vi "observacao.vi"() -> ()   [LabVIEW 2012] (continued)
            # "MUDANÇA:\nBit EMBREAGEM trocado pelos bits RAPIDO e LIGEIRO para detectar a retirada do objeto da posição centrada."
            # "MUDANÇA FUTURA:\nTrocar globais de calagem por valores \"latch\" dessas globais. Finalidade: manter display de coordenadas consistentes mesmo quando o usuário zerar as calagens, especialmente a local, para o próximo apontamento."
            # "ATUALIZA INDICADORES DO PAINEL"
            n267 = local read "ChkCalGlobal"() -> (w274:bool)
            n268 = global read "Global_Telescopio.vi" "PosDEC"() -> (w277:dbl)
            n269 = global read "Global_Telescopio.vi" "Sideral Time"() -> (w279:dbl)
            n270 = global read "Global_Telescopio.vi" "ObjCentrado"() -> (w250:bool)
            "ObjCentrado" <- w250
            n271 = global read "Global_Telescopio.vi" "PosAH"() -> (w278:dbl)
            n272 = call "Calcula epoch.vi"() -> ("epoch"=→"Epoch":dbl)  [unwired: 2 in]
            n273 = call "Bit Status AH.vi"("NomeStatus"=w263) -> ("StatBit"=w261:bool)
            n274 = call "Bit Status AH.vi"("NomeStatus"=w258) -> ("StatBit"=w257:bool)
            n275 = call "Bit Status DEC.vi"("NomeStatus"=w262) -> ("StatBit"=w255:bool)
            n276 = call "Bit Status DEC.vi"("NomeStatus"=w259) -> ("StatBit"=w256:bool)
            n277 = Compound Arithmetic op=OR(w261, w257, w255, w256) -> (w260:bool)
            n278 = case shown="True" w260 {
              frame False {
              }
              frame True {
                n279 = global write "Global_Telescopio.vi" "ObjCentrado"(FALSE) -> ()
              }
            }
            n280 = Tick Count (ms)() -> (millisecond timer value=w246:u32)
            n281 = local read "LedPointing"() -> (w245:bool)
            n282 = case shown="True" w250 {
              tunnel: [w356 w373] -> w271
              tunnel: [w355 w372] -> w267
              tunnel: [w358 w376] -> w251
              tunnel: [w357 w374] -> w264
              tunnel: w279 -> [w356 w373]
              tunnel: w278 -> [w361 _]
              tunnel: w277 -> [w360 _]
              tunnel: w274 -> [w359 _]
              tunnel: [w354 w370] -> _
              tunnel: w246 -> [w354 w370]
              frame False {
                n283 = case shown="False" w359 {
                  tunnel: w360 -> [w363 w369]
                  tunnel: [w363 w368] -> w358
                  tunnel: w361 -> [w362 w367]
                  tunnel: [w362 w364] -> w357
                  frame False {
                  }
                  frame True {
                    n284 = global read "Global_Telescopio.vi" "Calagem AH"() -> (w365:dbl)
                    n285 = global read "Global_Telescopio.vi" "Calagem DEC"() -> (w366:dbl)
                    n286 = Subtract(x=w367, y=w365) -> (x-y=w364:dbl)
                    n287 = Subtract(x=w369, y=w366) -> (x-y=w368:dbl)
                  }
                }
                n288 = Subtract(x=w356, y=w357) -> (x-y=w355:dbl)
              }
              frame True {
                # "PROCESSO PRECESSÃO"
                n289 = local read "Temp amb"() -> (w379:string)
                n290 = local read "hum local"() -> (w377:string)
                n291 = local read "MeanDEC"() -> (w380:string)
                n292 = local read "pressão atm"() -> (w378:string)
                n293 = local read "PM_RA"() -> (w375:string)
                n294 = local read "MeanRA"() -> (w381:string)
                n295 = local read "PM_DEC"() -> (w371:string)
                n296 = call "PrecessFortran.vi"("Asc reta"=w381, "Var RA"=w375, "Declinação"=w380, "Temperatura (Kelvin)"=w379, "Pressao atmosferica (mB)"=w378, "Humidade relativa (0 a 1)"=w377, "Var DEC"=w371) -> ("Observed RA (radians)"=w372:dbl, "Observed Dec (radians)"=w376:dbl)  [unwired: 2 in, 5 out]
                n297 = Subtract(x=w373, y=w372) -> (x-y=w374:dbl)
              }
            }
            "AtualDEC" <- w251
            n298 = case shown="True" w250 {
              tunnel: w251 -> [_ w310]
              tunnel: [w307 w309] -> w276
              tunnel: [w307 w308] -> w275
              frame False {
                w307 = 0.0
              }
              frame True {
                n299 = stacked-sequence {
                  seq-local: [w311 _ _] -> [_ _ w349]
                  tunnel: w310 -> [_ w318 _]
                  tunnel: [_ w317 _] -> w309
                  tunnel: [_ w316 _] -> w308
                  frame #0 {
                    n300 = Tick Count (ms)() -> (millisecond timer value=w311:u32)
                  }
                  frame #1 {
                    w319 = u16 3 items=["Alarme", "Atencao", "Erro", "Ocupado", "Protecao", "Embreagem", "Tracking", "Var. Track", "Rápido", "Ligeiro", "Médio", "Lento", "Em movimento", ""] ("NomeStatus")
                    w320 = u16 3 items=["Alarme", "Atencao", "Erro", "Ocupado", "Protecao", "Embreagem", "Tracking", "Var. Track", "Rápido", "Ligeiro", "Médio", "Lento", "Em movimento", ""] ("NomeStatus")
                    # "PROCESSO LEITURA POS_MOTOR"
                    n301 = local read "MOV_IDX_AH"() -> (w314:bool)
                    n302 = local read "MOV_IDX_DEC"() -> (w312:bool)
                    n303 = call "Bit Status AH.vi"("NomeStatus"=w320) -> ("StatBit"=w315:bool)
                    n304 = call "Bit Status DEC.vi"("NomeStatus"=w319) -> ("StatBit"=w313:bool)
                    n305 = case shown="False" w315 {
                      tunnel: w318 -> [w334 _]
                      tunnel: [w333 w348] -> w317
                      tunnel: w314 -> [w332 _]
                      frame False {
                        n306 = case shown="False" w332 {
                          tunnel: w334 -> [w342 _]
                          tunnel: [w338 w347] -> w333
                          frame False {
                            w345 = u16 1 items=["ZERO", "AH", "DEC", "TUBO", "CUP"] ("Controlador")
                            # "RA"
                            # "AH"
                            n307 = call "Get Posic Motor Indexer.vi"("Controlador"=w345) -> ("PosMotor"=w336:dbl)
                            n308 = global read "Global_Telescopio.vi" "AcumPrecRA"() -> (w339:dbl)
                            n309 = Negate(x=w336) -> (-x=w337:dbl)
                            n310 = Subtract(x=w337, y=w339) -> (x-y=w346:dbl)
                            n311 = global read "Global_Telescopio.vi" "AcumAG RA"() -> (w340:dbl)
                            n312 = Cosine(x=w342) -> (cos(x)=w341:dbl)
                            n313 = Absolute Value(x=w341) -> (abs(x)=w335:dbl)
                            n314 = Subtract(x=w346, y=w340) -> (x-y=w344:dbl)
                            n315 = Multiply(x=w335, y=w344) -> (x*y=w343:dbl)
                            n316 = call "Rad to Arcsec.vi"("Radiano"=w343) -> ("Arcsec"=w338:dbl)
                          }
                          frame True {
                            n317 = local read "Offset RA"() -> (w347:dbl)
                          }
                        }
                      }
                      frame True {
                        n318 = local read "Offset RA"() -> (w348:dbl)
                      }
                    }
                    n319 = case shown="False" w313 {
                      tunnel: [w322 w331] -> w316
                      tunnel: w312 -> [w321 _]
                      frame False {
                        n320 = case shown="False" w321 {
                          tunnel: [w323 w330] -> w322
                          frame False {
                            w326 = u16 2 items=["ZERO", "AH", "DEC", "TUBO", "CUP"] ("Controlador")
                            n321 = call "Get Posic Motor Indexer.vi"("Controlador"=w326) -> ("PosMotor"=w328:dbl)
                            n322 = global read "Global_Telescopio.vi" "AcumPrecDEC"() -> (w324:dbl)
                            n323 = Subtract(x=w328, y=w324) -> (x-y=w329:dbl)
                            n324 = global read "Global_Telescopio.vi" "AcumAG DEC"() -> (w325:dbl)
                            n325 = Subtract(x=w329, y=w325) -> (x-y=w327:dbl)
                            n326 = call "Rad to Arcsec.vi"("Radiano"=w327) -> ("Arcsec"=w323:dbl)
                          }
                          frame True {
                            n327 = local read "Offset DEC"() -> (w330:dbl)
                          }
                        }
                      }
                      frame True {
                        n328 = local read "Offset DEC"() -> (w331:dbl)
                      }
                    }
                  }
                  frame #2 {
                    n329 = flat-sequence {
                      tunnel: w349 -> [w350]
                      frame #0 {
                        n330 = Tick Count (ms)() -> (millisecond timer value=w351:u32)
                        n331 = Subtract(x=w351, y=w351) -> (x-y=→"dtAUX2":u32)
                        n332 = Subtract(x=w351, y=w350) -> (x-y=→"dtAUX3":u32)
                      }
                    }
                  }
                }
              }
            }
            "Offset RA" <- w276
            "Offset DEC" <- w275
            n333 = case shown="False" w245 {
              frame False {
                w285 = 0
                n334 = property on="BtPointPrecess" class="Bool"("DisabledEnum"=w285) -> ()  [unwired: 2 in, 2 out]
                n335 = property on="BtPointObjClear" class="Bool"("DisabledEnum"=w285) -> ()  [unwired: 2 in, 2 out]
              }
              frame True {
                w286 = 2
                n336 = property on="BtPointPrecess" class="Bool"("DisabledEnum"=w286) -> ()  [unwired: 2 in, 2 out]
                n337 = property on="BtPointObjClear" class="Bool"("DisabledEnum"=w286) -> ()  [unwired: 2 in, 2 out]
              }
            }
            n338 = call "Normliza_AH.vi"("PosAH"=w264) -> ("Numeric"=w249:dbl)
            n339 = Add(x=w269, y=w267) -> (x+y=w268:dbl)
            n340 = Add(x=w269, y=w271) -> (x+y=w272:dbl)
            n341 = Less Than 0?(x=w271) -> (x < 0?=w273:bool)
            n342 = Less Than 0?(x=w267) -> (x < 0?=w270:bool)
            n343 = Select(t=w272, s=w273, f=w271) -> (s? t:f=w252:dbl)
            n344 = Select(t=w268, s=w270, f=w267) -> (s? t:f=w253:dbl)
            n345 = case shown="True" w250 {
              tunnel: ["" w294] -> w254
              tunnel: w253 -> [_ w291]
              tunnel: w252 -> [_ w292]
              tunnel: w251 -> [_ w293]
              frame False {
              }
              frame True {
                n346 = disable-structure shown="Disabled" {
                  disable-tunnel: w293 -> [w305 _]
                  disable-tunnel: w292 -> [w304 _]
                  disable-tunnel: w291 -> [w303 _]
                  disable-tunnel: [w302 _] -> _
                  frame Disabled {
                    n347 = call "Hora_Limite.vi"("Asc Reta RA rad"=w303, "Sideral Time rad"=w304, "Declinação rad"=w305) -> ("TO Tempo de Observação Horas"=w302:dbl)  [unwired: 2 in]
                  }
                  frame Enabled {
                  }
                }
                n348 = call "Novo_tempo_obs.vi"() -> ("TO rad"=w289:dbl)  [unwired: 10 in, 1 out]
                n349 = Greater Than 0?(x=w289) -> (x > 0?=w288:bool)
                n350 = case shown="True" w288 {
                  tunnel: [w296 w299] -> w290
                  tunnel: w289 -> [w296 w298]
                  frame False {
                  }
                  frame True {
                    n351 = Random Number (0-1)() -> (number: 0 to 1=w300:dbl)
                    n352 = Multiply(x=w300, y=7.27e-05) -> (x*y=w297:dbl)
                    n353 = Add(x=w298, y=w297) -> (x+y=w299:dbl)
                  }
                }
                n354 = call "rad_hms.vi"("TRUE=HORA\nFALSE=GRAU"=TRUE ("TRUE=HORA\nFALSE=GRAU"), "Radiano"=w290) -> ("Hora/Graus Texto Decimal"=w294:string)  [unwired: 3 in]
              }
            }
            "Time to Limit" <- w254
            n355 = call "rad_hms.vi"("TRUE=HORA\nFALSE=GRAU"=TRUE ("TRUE=HORA\nFALSE=GRAU"), "Radiano"=w252) -> ("Hora/Graus Texto Decimal"=w266:string)  [unwired: 3 in]
            "Sideral time" <- w266
            n356 = call "rad_hms.vi"("TRUE=HORA\nFALSE=GRAU"=TRUE, "Radiano"=w253) -> ("Hora/Graus Texto Decimal"=w265:string)  [unwired: 3 in]
            "Right Ascention" <- w265
            n357 = call "rad_hms.vi"("TRUE=HORA\nFALSE=GRAU"=TRUE, "Radiano"=w249) -> ("Hora/Graus Texto Decimal"=w248:string)  [unwired: 3 in]
            "Hour Angle" <- w248
            "Hour Angle 2" <- w248
            n358 = call "rad_hms.vi"("TRUE=HORA\nFALSE=GRAU"=FALSE, "Radiano"=w251) -> ("Hora/Graus Texto Decimal"=w247:string)  [unwired: 3 in]
            "Declination" <- w247
            "DEC" <- w247
            n359 = global write "Global_Telescopio.vi" "Right Ascention"(w265) -> ()
            n360 = global write "Global_Telescopio.vi" "Hour Angle"(w248) -> ()
            n361 = global write "Global_Telescopio.vi" "Sideral time"(w266) -> ()
            n362 = global write "Global_Telescopio.vi" "Declination"(w247) -> ()
            n363 = global write "Global_Telescopio.vi" "AH_now"(w249) -> ()
            n364 = global write "Global_Telescopio.vi" "delta_now"(w251) -> ()
          }
          frame #2 {
            w406 = -0.39330025  # LatOPD rad
            # "ALTERAÇÃO FEITA EM 12/12/2012\nFEITA PARA RESOLVER EXCESSÍVOS\nMOVIMENTOS DO ACOMP.SID. DA\nCÚPULA (DANIEL). A condição de statCUP=0 foi inserida em 08/5/2013-> Só corrige a cúpula se esta estiver parada!"
            # "Horas"
            # "MUDANÇA FUTURA:\nPassar LatOPD para Global"
            # "az"
            # "z"
            # "Cálculo do Azimute da Cúpula e Hab Acompanham. Cúpula"
            # "Lógica de Segurança"
            # "ANGULO ZENITAL"
            n365 = global read "Global_Telescopio.vi" "OffsetCupula"() -> (w415:dbl)
            n366 = global read "Global_Telescopio.vi" "AH_now"() -> (w397:dbl)
            n367 = global read "Global_Telescopio.vi" "delta_now"() -> (w405:dbl)
            n368 = global read "Global_Telescopio.vi" "ErroMaxCup"() -> (w384:i16)
            n369 = global read "Global_Telescopio.vi" "Limite EAST"() -> (w398:dbl)
            n370 = global read "Global_Telescopio.vi" "Limite WEST"() -> (w399:dbl)
            n371 = global read "Global_Telescopio.vi" "PosCUP"() -> (w385:i16)
            "PosCUP" <- w385
            n372 = local read "Tick Cupula"() -> (w389:u32)
            n373 = call "Calculo_do_Azimute_da_Cupula_2.vi"("AH"=w397, "DEC"=w405, "OffsetTCSPD"=w415) -> ("PosCup"=w382:u16)  [unwired: 3 in, 1 out]
            "Azimute cup" <- w382
            n374 = Tick Count (ms)() -> (millisecond timer value=w390:u32)
            n375 = Multiply(x=w397, y=3.8197) -> (x*y=w400:dbl)
            n376 = call "Altura_e_Azimute.vi"("LAT rad"=w406, "DEC rad"=w405, "AH rad"=w397) -> ("AZIMUTE graus"=w403:dbl, "ANG. ZENITAL graus"=w404:dbl, "AZIMUTE rad"=w407:dbl, "ANG. ZENITAL rad"=w408:dbl)  [unwired: 2 out]
            "Azimuth" <- w403
            "Zenital angle" <- w404
            n377 = Greater Or Equal?(x=w390, y=w389) -> (x >= y?=w388:bool)
            n378 = Greater?(x=w400, y=w398) -> (0:w396:bool)
            n379 = Less?(x=w400, y=w399) -> (x < y?=w395:bool)
            n380 = call "Verifica_Correcao_CUP.vi"("Erro max"=w384, "Pos Atual"=w385, "Azimute"=w382) -> ("Corrigir?"=w383:bool)  [unwired: 2 in]
            n381 = Not And(1:w395, 2:w396) -> (0:w392:bool)
            n382 = local read "statCUP"() -> (w387:i32)
            n383 = call "Calcula_Proteção.vi"("Zenital angle rad"=w408, "Azimute rad"=w407) -> ("Z_SEGURANÇA_GRAUS"=w417:dbl, "Prot Segur"=w419:bool, "Z_LIBERA_GRAUS"=w416:dbl, "Z_MAX_GRAUS"=w418:dbl, "Prot Zmax"=w393:bool)
            n384 = Equal To 0?(x=w387) -> (x = 0?=w386:bool)
            n385 = global write "Global_Telescopio.vi" "Z_SEGURANÇA_GRAUS"(w417) -> ()
            n386 = global write "Global_Telescopio.vi" "Zenital angle GRAUS"(w404) -> ()
            n387 = global write "Global_Telescopio.vi" "Azimute GRAUS"(w403) -> ()
            n388 = global write "Global_Telescopio.vi" "Z_MAX_GRAUS"(w418) -> ()
            n389 = global write "Global_Telescopio.vi" "Z_LIBERA_GRAUS"(w416) -> ()
            n390 = Compound Arithmetic op=AND(w383, "DOME", w388, w386) -> (w414:bool)
            n391 = case shown="True" w414 {
              tunnel: w382 -> [_ w428]
              tunnel: FALSE -> [_ w426]
              frame False {
              }
              frame True {
                # "TEMPO CÚPULA"
                # "2m Tempo para novo movimento"
                n392 = local write "Dome on Target"(w426) -> ()
                n393 = Tick Count (ms)() -> (millisecond timer value=w425:u32)
                n394 = To Word Integer(number=w428) -> (16bit integer=w422:i16)
                n395 = local write "statCUP"(1 ("statCUP")) -> ()
                n396 = Add(x=w425, y=u32 120000) -> (x+y=→"Tick Cupula":u32)
                n397 = global write "Global_Telescopio.vi" "TargetCUP"(w422) -> ()
              }
            }
            n398 = Or(x=w392, y=w393) -> (x .or. y?=w394:bool)
            n399 = global read "Global_Telescopio.vi" "LIMITE"() -> (w413:bool)
            n400 = Or(x=w413, y=w394) -> (x .or. y?=w412:bool)
            "Proteção" <- w412
            n401 = call "Borda_Subida_Segurança.vi"("Entrada"=w419) -> ("Boolean"=w420:bool)
            n402 = call "Borda_Subida_Z_max.vi"("Entrada"=w412) -> ("Boolean"=w421:bool)
            n403 = Select(t=u8 2 ("Disabled"), s=w412, f=u8 0 ("Disabled")) -> (s? t:f=w409:u8)
            n404 = property on="MOUNT" class="Bool (strict)"("Disabled"=w409) -> ()  [unwired: 2 in, 2 out]
            n405 = case shown="True" w420 {
              frame False {
              }
              frame True {
                w431 = u16 2 items=["ZERO", "AH", "DEC", "TUBO", "CUP"] ("Controlador")
                w430 = "FREAR" ("Comando")
                w432 = u16 1 items=["ZERO", "AH", "DEC", "TUBO", "CUP"] ("Controlador")
                w429 = "EIXO" ("Dispositivo")
                n406 = call "Monta Comando.vi"("Comando"=w430, "Dispositivo"=w429, "Controlador"=w432) -> ()  [unwired: 4 in, 3 out]
                n407 = call "Monta Comando.vi"("Comando"=w430, "Dispositivo"=w429, "Controlador"=w431) -> ()  [unwired: 4 in, 3 out]
              }
            }
            n408 = case shown="True" w421 {
              frame False {
              }
              frame True {
                w435 = FALSE
                w433 = "Telescópio parado por inclinação excessiva!" ("SYSTEM MESSAGES")
                n409 = local write "LED MOUNT"(w435) -> ()
                n410 = local write "MOUNT"(w435) -> ()
                n411 = global write "Global_Telescopio.vi" "ObjCentrado"(FALSE) -> ()
                n412 = global write "Global_Telescopio.vi" "STOP ALL"(TRUE ("STOP ALL")) -> ()
                n413 = call "Monta_Mensagem.vi"("Mensagem"=w433) -> ()  [unwired: 2 in]
                n414 = call "Salva_systems_messages.vi"("Mensagem"=w433) -> ()  [unwired: 5 in]
              }
            }
            "Led Chave Dome" <- "DOME"
          }
          frame #3 {
            w442 = u32 500 ("millisecond multiple")
            w456 = u16 3 items=["Alarme", "Atencao", "Erro", "Ocupado", "TBD", "LCB", "Trapeira", "Paravento", "DomoRap", "DomoCW", "DomoCCW", "TBD", "Em movimento", "TBD"] ("NomeStatus")
            w470 = u16 3 items=["Alarme", "Atencao", "Erro", "Ocupado", "Protecao", "Embreagem", "Tracking", "Var. Track", "Rápido", "Ligeiro", "Médio", "Lento", "Em movimento", ""] ("NomeStatus")
            w471 = u16 3 items=["Alarme", "Atencao", "Erro", "Ocupado", "Protecao", "Embreagem", "Tracking", "Var. Track", "Rápido", "Ligeiro", "Médio", "Lento", "Em movimento", ""] ("NomeStatus")
            # "04-07-2022\nValor de Erro PROTEC\nalterado de 5 para 10"
            # "MUDANÇA: \nIncluído CASE"
            # "Esse metrônomo determina\no ciclo de 0,5 segundo dos\ncálculos rápidos e totais!"
            # "PROCESSO APONTAMENTO"
            # "MÁQUINA DE ESTADO DO APONTAMENTO"
            # "Seta nome para GO/STOP"
            n415 = global read "Global_Telescopio.vi" "LimiarRapMed"() -> (w472:dbl)
            n416 = global write "Global_Telescopio.vi" "Estado DEC"("statDEC") -> ()
            n417 = global read "Global_Telescopio.vi" "Sideral Time"() -> (w450:dbl)
            n418 = global read "Global_Telescopio.vi" "PosAH"() -> (w475:dbl)
            n419 = global read "Global_Telescopio.vi" "ErroMaxEixo"() -> (w459:dbl)
            n420 = global read "Global_Telescopio.vi" "PosDEC"() -> (w473:dbl)
            n421 = global read "Global_Telescopio.vi" "TargetRA"() -> (w476:dbl)
            n422 = global read "Global_Telescopio.vi" "TargetDEC"() -> (w474:dbl)
            n423 = call "Bit Status DEC.vi"("NomeStatus"=w470) -> ("StatBit"=w458:bool)
            n424 = call "Bit Status AH.vi"("NomeStatus"=w471) -> ("StatBit"=w457:bool)
            n425 = case shown="4" "statDEC" {
              selector: "statDEC" -> [w605 _ _ _ _ _ _ _ _]
              tunnel: [w605 w612 w642 w664 w691 w715 0 ("t") w732 w737] -> w451
              tunnel: w474 -> [_ w611 _ w658 _ _ _ _ _]
              tunnel: w473 -> [_ w607 _ w661 _ _ _ _ _]
              tunnel: w459 -> [_ _ _ w662 _ _ _ _ _]
              tunnel: w472 -> [_ w613 _ _ _ _ _ _ _]
              tunnel: w458 -> [_ w610 _ w657 _ _ _ _ _]
              frame 0, Default {
                w603 = 0 ("CR DEC")
                # "Sem apontamento"
                n426 = call "TickTimeout.vi"() -> ("msTick"=→"TimeoutDEC":u32)  [unwired: 2 in, 2 out]
                n427 = local write "CR DEC"(w603) -> ()
                n428 = local write "C. DEC"(w603) -> ()
              }
              frame 1 {
                # "Envia\nComando"
                n429 = Subtract(x=w611, y=w607) -> (x-y=w609:dbl)
                n430 = Absolute Value(x=w609) -> (abs(x)=w614:dbl)
                n431 = Less?(x=w614, y=w613) -> (x < y?=w608:bool)
                n432 = case shown="False" w608 {
                  tunnel: [w618 3] -> w612
                  tunnel: w611 -> [w617 _]
                  tunnel: w609 -> [w616 _]
                  tunnel: w610 -> [w615 _]
                  frame False {
                    # "destino"
                    # "Fora do"
                    n433 = case shown="False" w615 {
                      tunnel: [w622 w630] -> w618
                      tunnel: w617 -> [w625 _]
                      tunnel: w616 -> [_ _]
                      frame False {
                        w629 = u16 2 items=["ZERO", "AH", "DEC", "TUBO", "CUP"] ("Controlador")
                        # "limpa flag"
                        # "CLP Pronto"
                        n434 = local write "Flag ativo DEC"(FALSE ("Flag ativo DEC")) -> ()
                        n435 = call "rad_hms.vi"("TRUE=HORA\nFALSE=GRAU"=FALSE, "Radiano"=w625) -> ("Hora/Graus Texto Decimal"=w626:string)  [unwired: 3 in]
                        n436 = call "Monta Comando.vi"("Set Point"=w626, "Comando"="MOVER_RAP", "Dispositivo"="EIXO" ("Comando"), "Controlador"=w629) -> ("Erro Comunicação"=w620:bool)  [unwired: 3 in, 2 out]
                        n437 = Select(t=6, s=w620, f=20) -> (s? t:f=w622:i32)
                      }
                      frame True {
                        # "CLP Ocupado"
                        n438 = local read "TimeoutDEC"() -> (w632:u32)
                        n439 = call "TickTimeout.vi"("msInicial"=w632, "msTimeout"=u32 4000) -> ("Timeout"=w631:bool)  [unwired: 2 out]
                        n440 = case shown="False" w631 {
                          tunnel: [1 5] -> w630
                          frame False {
                          }
                          frame True {
                            # "Tratar\nTimeout"
                          }
                        }
                      }
                    }
                  }
                  frame True {
                    # "Dist. pequena p/ mov. rápido"
                    # "Ligar mov. lento"
                    n441 = call "TickTimeout.vi"() -> ("msTick"=w636:u32)  [unwired: 2 in, 2 out]
                    n442 = local write "TimeoutDEC"(w636) -> ()
                  }
                }
                n443 = local write "dec="(FALSE ("dec=")) -> ()
              }
              frame 2 {
                w643 = u16 12 items=["Alarme", "Atencao", "Erro", "Ocupado", "Protecao", "Embreagem", "Tracking", "Var. Track", "Rápido", "Ligeiro", "Médio", "Lento", "Em movimento", ""] ("NomeStatus")
                # "Aguarda fim mov. Rap."
                n444 = call "Bit Status DEC.vi"("NomeStatus"=w643) -> ("StatBit"=w644:bool)
                n445 = case shown="True" w644 {
                  tunnel: [1 w653] -> w641
                  frame False {
                    # "Motor parado.\nTestar se chegou\nao destino"
                    n446 = call "TickTimeout.vi"() -> ("msTick"=w649:u32)  [unwired: 2 in, 2 out]
                    n447 = local write "TimeoutDEC"(w649) -> ()
                  }
                  frame True {
                    # "Ainda movendo...\nAGUARDAR"
                    n448 = local read "Erro PROTEC"() -> (w655:i32)
                    n449 = call "PROTECAO_DEC.vi"() -> ("CONT DEC"=w656:i32)  [unwired: 11 in]
                    "C. DEC" <- w656
                    n450 = Greater Or Equal?(x=w656, y=w655) -> (x >= y?=w651:bool)
                    n451 = Select(t=6, s=w651, f=2) -> (s? t:f=w653:i32)
                  }
                }
                n452 = global read "Global_Telescopio.vi" "Habilita supervisao"() -> (w639:bool)
                n453 = case shown="True" w639 {
                  tunnel: [FALSE w648] -> w638
                  frame False {
                  }
                  frame True {
                    n454 = local read "Erro Lim"() -> (w646:i32)
                    n455 = Greater Or Equal?(x="CR DEC", y=w646) -> (x >= y?=w648:bool)
                  }
                }
                n456 = Select(t=6, s=w638, f=w641) -> (s? t:f=w642:i32)
              }
              frame 3 {
                # "Mov.Lento"
                n457 = Subtract(x=w658, y=w661) -> (x-y=w659:dbl)
                n458 = Absolute Value(x=w659) -> (abs(x)=w663:dbl)
                n459 = Less Or Equal?(x=w663, y=w662) -> (x <= y?=w660:bool)
                n460 = case shown="False" w660 {
                  selector: w660 -> [_ w687]
                  tunnel: [w666 0] -> w664
                  tunnel: w659 -> [w665 _]
                  tunnel: w658 -> [_ w686]
                  tunnel: w657 -> [w667 _]
                  frame False {
                    n461 = case shown="False" w667 {
                      tunnel: [w671 w680] -> w666
                      tunnel: w665 -> [w674 _]
                      frame False {
                        w679 = u16 2 items=["ZERO", "AH", "DEC", "TUBO", "CUP"] ("Controlador")
                        # "limpa flag"
                        # "Mov. lento"
                        n462 = call "TickTimeout.vi"() -> ("msTick"=w673:u32)  [unwired: 2 in, 2 out]
                        n463 = local write "TimeoutDEC"(w673) -> ()
                        n464 = call "rad_hms.vi"("TRUE=HORA\nFALSE=GRAU"=FALSE ("TRUE=HORA\nFALSE=GRAU"), "Radiano"=w674) -> ("Hora/Graus Texto Decimal"=w676:string)  [unwired: 3 in]
                        n465 = local write "Flag ativo DEC"(FALSE ("Flag ativo DEC")) -> ()
                        n466 = call "Monta Comando.vi"("Set Point"=w676, "Comando"="MOVER_REL", "Dispositivo"="EIXO" ("Comando"), "Controlador"=w679) -> ("Erro Comunicação"=w669:bool)  [unwired: 3 in, 2 out]
                        n467 = Select(t=6, s=w669, f=40) -> (s? t:f=w671:i32)
                      }
                      frame True {
                        # "CLP Ocupado"
                        n468 = local read "TimeoutDEC"() -> (w682:u32)
                        n469 = call "TickTimeout.vi"("msInicial"=w682, "msTimeout"=u32 2000) -> ("Timeout"=w681:bool)  [unwired: 2 out]
                        n470 = case shown="False" w681 {
                          tunnel: [3 5] -> w680
                          frame False {
                          }
                          frame True {
                          }
                        }
                      }
                    }
                  }
                  frame True {
                    # "DEC no destino"
                    n471 = local write "LatchDeslocDEC"(w686) -> ()
                    "DEC on Target" <- w687
                  }
                }
              }
              frame 4 {
                w694 = u16 12 items=["Alarme", "Atencao", "Erro", "Ocupado", "Protecao", "Embreagem", "Tracking", "Var. Track", "Rápido", "Ligeiro", "Médio", "Lento", "Em movimento", ""] ("NomeStatus")
                # "Aguarda fim mov. lento"
                n472 = call "Bit Status DEC.vi"("NomeStatus"=w694) -> ("StatBit"=w695:bool)
                n473 = case shown="True" w695 {
                  tunnel: [3 w705] -> w690
                  frame False {
                    # "Motor parado.\nTestar se chegou\nao destino"
                    n474 = call "TickTimeout.vi"() -> ("msTick"=w700:u32)  [unwired: 2 in, 2 out]
                    n475 = local write "TimeoutDEC"(w700) -> ()
                  }
                  frame True {
                    n476 = local read "Erro PROTEC"() -> (w707:i32)
                    n477 = call "PROTECAO_DEC.vi"() -> ("CONT DEC"=w702:i32)  [unwired: 11 in]
                    n478 = local write "C. DEC"(w702) -> ()
                    n479 = Greater Or Equal?(x=w702, y=w707) -> (x >= y?=w704:bool)
                    n480 = local read "TimeoutDEC"() -> (w709:u32)
                    n481 = call "TickTimeout.vi"("msInicial"=w709, "msTimeout"=u32 4000) -> ("Timeout"=w708:bool)  [unwired: 2 out]
                    n482 = case shown="False" w708 {
                      tunnel: [4 5] -> w703
                      frame False {
                      }
                      frame True {
                      }
                    }
                    n483 = Select(t=6, s=w704, f=w703) -> (s? t:f=w705:i32)
                  }
                }
                n484 = global read "Global_Telescopio.vi" "Habilita supervisao"() -> (w692:bool)
                n485 = case shown="True" w692 {
                  tunnel: [FALSE w699] -> w689
                  frame False {
                  }
                  frame True {
                    n486 = local read "CR DEC"() -> (w698:i32)
                    n487 = local read "Erro Lim"() -> (w697:i32)
                    n488 = Greater Or Equal?(x=w698, y=w697) -> (x >= y?=w699:bool)
                  }
                }
                n489 = Select(t=6, s=w689, f=w690) -> (s? t:f=w691:i32)
              }
              frame 5 {
                w720 = u16 2 items=["ZERO", "AH", "DEC", "TUBO", "CUP"] ("Controlador")
                # "Reiniciar apontamento"
                # "Trata Timeout"
                n490 = call "TickTimeout.vi"() -> ("msTick"=w717:u32)  [unwired: 2 in, 2 out]
                n491 = local write "TimeoutDEC"(w717) -> ()
                n492 = call "Monta Comando.vi"("Comando"="PARAR", "Dispositivo"="PROG" ("Comando"), "Controlador"=w720) -> ("Erro Comunicação"=w713:bool)  [unwired: 4 in, 2 out]
                n493 = Select(t=6, s=w713, f=1) -> (s? t:f=w715:i32)
              }
              frame 6 {
                # "PARADA POR ERRO DO CONTROLADOR"
                n494 = stacked-sequence {
                  frame #0 {
                    w723 = u16 2 items=["ZERO", "AH", "DEC", "TUBO", "CUP"] ("Controlador")
                    n495 = call "Monta Comando.vi"("Comando"="PARAR", "Dispositivo"="PROG" ("Comando"), "Controlador"=w723) -> ()  [unwired: 4 in, 3 out]
                    "dec=" <- TRUE ("ah=")
                  }
                  frame #1 {
                    w726 = "Erro de Controlador DEC , REAPONTAR !" ("Mensagem")
                    n496 = local write "Flag de erro p/ apagar lampada"(TRUE ("Flag de erro p/ apagar lampada")) -> ()
                    n497 = call "Monta_Mensagem.vi"("Mensagem"=w726) -> ()  [unwired: 2 in]
                    n498 = call "Salva_systems_messages.vi"("Mensagem"=w726) -> ()  [unwired: 5 in]
                  }
                  frame #2 {
                    w729 = u16 2 items=["ZERO", "AH", "DEC", "TUBO", "CUP"] ("Controlador")
                    # "Em movimento não aceita reset"
                    # "Segundo PARAR por garantia"
                    n499 = call "Monta Comando.vi"("Comando"="PARAR", "Dispositivo"="PROG", "Controlador"=w729) -> ()  [unwired: 4 in, 3 out]
                  }
                }
              }
              frame 20 {
                # "Espera entrar\nem movimento"
                n500 = local read "Flag ativo DEC"() -> (w731:bool)
                n501 = case shown="True" w731 {
                  tunnel: [20 ("t") 2 ("t")] -> w732
                  frame False {
                  }
                  frame True {
                    # "limpa flag"
                    n502 = local write "Flag ativo DEC"(FALSE ("Flag ativo AH")) -> ()
                  }
                }
              }
              frame 40 {
                # "Espera entrar\nem movimento"
                n503 = local read "Flag ativo DEC"() -> (w736:bool)
                n504 = case shown="True" w736 {
                  tunnel: [40 ("t") 4 ("t")] -> w737
                  frame False {
                  }
                  frame True {
                    # "limpa flag"
                    n505 = local write "Flag ativo DEC"(FALSE ("Flag ativo AH")) -> ()
                  }
                }
              }
            }
            n506 = global write "Global_Telescopio.vi" "Estado AH"("statAH") -> ()
            n507 = case shown="1" "statAH" {
              selector: "statAH" -> [w743 _ _ _ _ _ _ _ _ _]
              tunnel: [w743 w752 w780 w796 w820 w848 w873 0 ("t") w889 w894] -> w455
              tunnel: w450 -> [_ w749 _ _ w817 _ _ _ _ _]
              tunnel: w476 -> [_ w748 _ _ w814 _ _ _ _ _]
              tunnel: w475 -> [_ w746 _ _ w816 _ _ _ _ _]
              tunnel: w459 -> [_ _ _ _ w821 _ _ _ _ _]
              tunnel: w472 -> [_ w753 _ _ _ _ _ _ _ _]
              tunnel: w457 -> [_ w750 _ w797 w818 _ _ _ _ _]
              frame 0, Default {
                w741 = 0 ("CR AH")
                # "Sem apontamento"
                n508 = call "TickTimeout.vi"() -> ("msTick"=→"TimeoutAH":u32)  [unwired: 2 in, 2 out]
                n509 = local write "CR AH"(w741) -> ()
                n510 = local write "C. AH"(w741) -> ()
              }
              frame 1 {
                # "Mov.Rapido"
                n511 = call "Calculo_AH.vi"("AH_Telescopio"=w746, "RA_Destino"=w748, "Hora Sideral"=w749) -> ("Dif_Abs_AH"=w747:dbl, "AH_Destino"=w744:dbl)  [unwired: 1 out]
                "AH_Destino" <- w744
                n512 = Less?(x=w747, y=w753) -> (x < y?=w751:bool)
                n513 = case shown="False" w751 {
                  tunnel: w744 -> [w754 _]
                  tunnel: [w755 3] -> w752
                  tunnel: w750 -> [w756 _]
                  frame False {
                    n514 = case shown="True" w756 {
                      tunnel: w754 -> [w762 _]
                      tunnel: [w759 w768] -> w755
                      frame False {
                        w764 = u16 1 items=["ZERO", "AH", "DEC", "TUBO", "CUP"] ("Controlador")
                        # "limpa flag"
                        # "Aguardar\nfim mov."
                        # "Mov. rápido"
                        n515 = local write "Flag ativo AH"(FALSE ("Flag ativo AH")) -> ()
                        n516 = call "rad_hms.vi"("TRUE=HORA\nFALSE=GRAU"=TRUE ("TRUE=HORA\nFALSE=GRAU"), "Radiano"=w762) -> ("Hora/Graus Texto Decimal"=w767:string)  [unwired: 3 in]
                        n517 = call "Monta Comando.vi"("Set Point"=w767, "Comando"="MOVER_RAP", "Dispositivo"="EIXO" ("Comando"), "Controlador"=w764) -> ("Erro Comunicação"=w761:bool)  [unwired: 3 in, 2 out]
                        n518 = Select(t=7, s=w761, f=20) -> (s? t:f=w759:i32)
                      }
                      frame True {
                        # "CLP Ocupado"
                        n519 = local read "TimeoutAH"() -> (w770:u32)
                        n520 = call "TickTimeout.vi"("msInicial"=w770, "msTimeout"=u32 8000) -> ("Timeout"=w769:bool)  [unwired: 2 out]
                        n521 = case shown="True" w769 {
                          tunnel: [1 6] -> w768
                          frame False {
                          }
                          frame True {
                            # "Tratar\nTimeout"
                          }
                        }
                      }
                    }
                  }
                  frame True {
                    # "Ligar acomp. sideral"
                    # "Dist. pequena p/ mov. rápido"
                    n522 = call "TickTimeout.vi"() -> ("msTick"=w774:u32)  [unwired: 2 in, 2 out]
                    n523 = local write "TimeoutAH"(w774) -> ()
                  }
                }
                n524 = local write "ah="(FALSE ("ah=")) -> ()
              }
              frame 2 {
                w782 = u16 12 items=["Alarme", "Atencao", "Erro", "Ocupado", "Protecao", "Embreagem", "Tracking", "Var. Track", "Rápido", "Ligeiro", "Médio", "Lento", "Em movimento", ""] ("NomeStatus")
                # "Aguarda fim mov. Rap."
                n525 = call "Bit Status AH.vi"("NomeStatus"=w782) -> ("StatBit"=w781:bool)
                n526 = case shown="True" w781 {
                  tunnel: [1 w791] -> w779
                  frame False {
                    # "Motor parado.\nTestar se precisa\nde novo cmd. \nde mov. rápido"
                    n527 = call "TickTimeout.vi"() -> ("msTick"=w787:u32)  [unwired: 2 in, 2 out]
                    n528 = local write "TimeoutAH"(w787) -> ()
                  }
                  frame True {
                    # "Aqui também \ncaberia um \nTimeout?"
                    # "Ainda movendo...\nAGUARDAR"
                    n529 = local read "AH_Destino"() -> (w789:dbl)
                    n530 = local read "Erro PROTEC"() -> (w795:i32)
                    n531 = call "PROTECAO_AH.vi"("AH_Destino"=w789) -> ("CONT AH"=w790:i32)  [unwired: 10 in]
                    "C. AH" <- w790
                    n532 = Greater Or Equal?(x=w790, y=w795) -> (x >= y?=w794:bool)
                    n533 = Select(t=7, s=w794, f=2) -> (s? t:f=w791:i32)
                  }
                }
                n534 = global read "Global_Telescopio.vi" "Habilita supervisao"() -> (w777:bool)
                n535 = case shown="True" w777 {
                  tunnel: [FALSE w785] -> w776
                  frame False {
                  }
                  frame True {
                    n536 = local read "Erro Lim"() -> (w784:i32)
                    n537 = Greater Or Equal?(x="CR AH", y=w784) -> (x >= y?=w785:bool)
                  }
                }
                n538 = Select(t=7, s=w776, f=w779) -> (s? t:f=w780:i32)
              }
              frame 3 {
                # "Liga Acomp. Sideral"
                n539 = case shown="True" w797 {
                  tunnel: [w798 w807] -> w796
                  frame False {
                    w802 = TRUE
                    w804 = u16 1 items=["ZERO", "AH", "DEC", "TUBO", "CUP"] ("Controlador")
                    # "Usar mov. lento"
                    # "CLP Pronto - Liga sideral"
                    n540 = call "Monta Comando.vi"("Comando"="LIGAR", "Dispositivo"="SIDERAL" ("Comando"), "Controlador"=w804) -> ("Erro Comunicação"=w800:bool)  [unwired: 4 in, 2 out]
                    n541 = Select(t=7, s=w800, f=4) -> (s? t:f=w798:i32)
                    n542 = call "TickTimeout.vi"() -> ("msTick"=w803:u32)  [unwired: 2 in, 2 out]
                    n543 = local write "LED MOUNT"(w802) -> ()
                    n544 = local write "MOUNT"(w802) -> ()
                    n545 = local write "TimeoutAH"(w803) -> ()
                  }
                  frame True {
                    # "CLP Ocupado"
                    n546 = local read "TimeoutAH"() -> (w809:u32)
                    n547 = call "TickTimeout.vi"("msInicial"=w809, "msTimeout"=u32 8000) -> ("Timeout"=w808:bool)  [unwired: 2 out]
                    n548 = case shown="True" w808 {
                      tunnel: [3 6] -> w807
                      frame False {
                      }
                      frame True {
                        # "Tratar\nTimeout"
                      }
                    }
                  }
                }
              }
              frame 4 {
                # "Mov.Lento"
                n549 = call "Calculo_AH.vi"("AH_Telescopio"=w816, "RA_Destino"=w814, "Hora Sideral"=w817) -> ("Dif_AH"=w813:dbl, "Dif_Abs_AH"=w815:dbl)  [unwired: 1 out]
                n550 = Less?(x=w815, y=w821) -> (x < y?=w819:bool)
                n551 = case shown="False" w819 {
                  selector: w819 -> [_ w844]
                  tunnel: [w823 0] -> w820
                  tunnel: w818 -> [w824 _]
                  tunnel: w814 -> [_ w843]
                  tunnel: w813 -> [w822 _]
                  frame False {
                    n552 = case shown="True" w824 {
                      tunnel: [w827 w837] -> w823
                      tunnel: w822 -> [w831 _]
                      frame False {
                        w833 = u16 1 items=["ZERO", "AH", "DEC", "TUBO", "CUP"] ("Controlador")
                        # "limpa flag"
                        # "Envia Cmd. Mov. Lento"
                        n553 = call "TickTimeout.vi"() -> ("msTick"=w830:u32)  [unwired: 2 in, 2 out]
                        n554 = local write "TimeoutAH"(w830) -> ()
                        n555 = local write "Flag ativo AH"(FALSE ("Flag ativo AH")) -> ()
                        n556 = call "rad_hms.vi"("TRUE=HORA\nFALSE=GRAU"=TRUE ("TRUE=HORA\nFALSE=GRAU"), "Radiano"=w831) -> ("Hora/Graus Texto Decimal"=w836:string)  [unwired: 3 in]
                        n557 = call "Monta Comando.vi"("Set Point"=w836, "Comando"="MOVER_REL", "Dispositivo"="EIXO" ("Comando"), "Controlador"=w833) -> ("Erro Comunicação"=w826:bool)  [unwired: 3 in, 2 out]
                        n558 = Select(t=7, s=w826, f=50) -> (s? t:f=w827:i32)
                      }
                      frame True {
                        # "CLP Ocupado"
                        n559 = local read "TimeoutAH"() -> (w839:u32)
                        n560 = call "TickTimeout.vi"("msInicial"=w839, "msTimeout"=u32 8000) -> ("Timeout"=w838:bool)  [unwired: 2 out]
                        n561 = case shown="False" w838 {
                          tunnel: [4 6] -> w837
                          frame False {
                          }
                          frame True {
                          }
                        }
                      }
                    }
                  }
                  frame True {
                    # "AH on Target"
                    n562 = local write "LatchDeslocRA"(w843) -> ()
                    "RA on Target" <- w844
                  }
                }
              }
              frame 5 {
                w852 = u16 12 items=["Alarme", "Atencao", "Erro", "Ocupado", "Protecao", "Embreagem", "Tracking", "Var. Track", "Rápido", "Ligeiro", "Médio", "Lento", "Em movimento", ""] ("NomeStatus")
                # "Aguarda fim mov. Lento"
                n563 = call "Bit Status AH.vi"("NomeStatus"=w852) -> ("StatBit"=w851:bool)
                n564 = case shown="True" w851 {
                  tunnel: [4 w864] -> w846
                  frame False {
                    # "Motor parado.\nTestar se chegou\nao destino"
                    n565 = call "TickTimeout.vi"() -> ("msTick"=w857:u32)  [unwired: 2 in, 2 out]
                    n566 = local write "TimeoutAH"(w857) -> ()
                  }
                  frame True {
                    # "Trata Timeout"
                    n567 = local read "AH_Destino"() -> (w859:dbl)
                    n568 = local read "Erro PROTEC"() -> (w862:i32)
                    n569 = call "PROTECAO_AH.vi"("AH_Destino"=w859) -> ("CONT AH"=w860:i32)  [unwired: 10 in]
                    n570 = local read "TimeoutAH"() -> (w867:u32)
                    n571 = Greater Or Equal?(x=w860, y=w862) -> (x >= y?=w861:bool)
                    n572 = local write "C. AH"(w860) -> ()
                    n573 = call "TickTimeout.vi"("msInicial"=w867, "msTimeout"=u32 8000) -> ("Timeout"=w866:bool)  [unwired: 2 out]
                    n574 = case shown="False" w866 {
                      tunnel: [5 6] -> w863
                      frame False {
                      }
                      frame True {
                        # "Tratar\nTimeout"
                      }
                    }
                    n575 = Select(t=7, s=w861, f=w863) -> (s? t:f=w864:i32)
                  }
                }
                n576 = global read "Global_Telescopio.vi" "Habilita supervisao"() -> (w850:bool)
                n577 = case shown="True" w850 {
                  tunnel: [FALSE w856] -> w847
                  frame False {
                  }
                  frame True {
                    n578 = local read "Erro Lim"() -> (w854:i32)
                    n579 = local read "CR AH"() -> (w855:i32)
                    n580 = Greater Or Equal?(x=w855, y=w854) -> (x >= y?=w856:bool)
                  }
                }
                n581 = Select(t=7, s=w847, f=w846) -> (s? t:f=w848:i32)
              }
              frame 6 {
                w876 = u16 1 items=["ZERO", "AH", "DEC", "TUBO", "CUP"] ("Controlador")
                # "Reiniciar apontamento"
                # "Trata Timeout"
                n582 = call "TickTimeout.vi"() -> ("msTick"=w875:u32)  [unwired: 2 in, 2 out]
                n583 = call "Monta Comando.vi"("Comando"="PARAR", "Dispositivo"="PROG" ("Comando"), "Controlador"=w876) -> ("Erro Comunicação"=w871:bool)  [unwired: 4 in, 2 out]
                n584 = local write "TimeoutAH"(w875) -> ()
                n585 = Select(t=7, s=w871, f=1) -> (s? t:f=w873:i32)
              }
              frame 7 {
                # "PARADA POR ERRO DO CONTROLADOR"
                n586 = stacked-sequence {
                  frame #0 {
                    w881 = u16 1 items=["ZERO", "AH", "DEC", "TUBO", "CUP"] ("Controlador")
                    n587 = call "Monta Comando.vi"("Comando"="PARAR", "Dispositivo"="PROG" ("Comando"), "Controlador"=w881) -> ()  [unwired: 4 in, 3 out]
                    "ah=" <- TRUE ("ah=")
                  }
                  frame #1 {
                    w884 = "Erro de Controlador RA , REAPONTAR !" ("Mensagem")
                    n588 = call "Monta_Mensagem.vi"("Mensagem"=w884) -> ()  [unwired: 2 in]
                    n589 = call "Salva_systems_messages.vi"("Mensagem"=w884) -> ()  [unwired: 5 in]
                    "Flag de erro p/ apagar lampada" <- TRUE ("Flag de erro p/ apagar lampada")
                  }
                  frame #2 {
                    w888 = u16 1 items=["ZERO", "AH", "DEC", "TUBO", "CUP"] ("Controlador")
                    # "Em movimento não aceita reset"
                    # "Segundo PARAR por garantia"
                    n590 = call "Monta Comando.vi"("Comando"="PARAR", "Dispositivo"="PROG", "Controlador"=w888) -> ()  [unwired: 4 in, 3 out]
                  }
                }
              }
              frame 20 {
                # "Espera entrar\nem movimento"
                n591 = local read "Flag ativo AH"() -> (w890:bool)
                n592 = case shown="True" w890 {
                  tunnel: [20 ("t") 2 ("t")] -> w889
                  frame False {
                  }
                  frame True {
                    # "limpa flag"
                    n593 = local write "Flag ativo AH"(FALSE ("Flag ativo AH")) -> ()
                  }
                }
              }
              frame 50 {
                # "Espera entrar\nem movimento"
                n594 = local read "Flag ativo AH"() -> (w895:bool)
                n595 = case shown="True" w895 {
                  tunnel: [50 ("t") 5 ("t")] -> w894
                  frame False {
                  }
                  frame True {
                    # "limpa flag"
                    n596 = local write "Flag ativo AH"(FALSE ("Flag ativo AH")) -> ()
                  }
                }
              }
            }
            n597 = call "PROTECAO.vi"("Estado In"=w451) -> ("Estado Out"=w437:i32)  [unwired: 2 in]
            n598 = local write "statDEC"(w437) -> ()
            n599 = local read "statCUP"() -> (w461:i32)
            n600 = local read "statDEC"() -> (w462:i32)
            n601 = local read "statAH"() -> (w463:i32)
            n602 = call "PROTECAO.vi"("Estado In"=w455) -> ("Estado Out"=w454:i32)  [unwired: 2 in]
            n603 = global read "Global_Telescopio.vi" "Botão GO = STOP"() -> (w449:bool)
            n604 = local write "statAH"(w454) -> ()
            n605 = Compound Arithmetic op=ADD(w461, w463, w462) -> (w465:i32)
            n606 = call "Bit Status CUP.vi"("NomeStatus"=w456) -> ("StatBit"=w469:bool)
            n607 = global read "Global_Telescopio.vi" "PosCUP"() -> (w468:i16)
            n608 = global read "Global_Telescopio.vi" "ErroMaxCup"() -> (w466:i16)
            n609 = global read "Global_Telescopio.vi" "TargetCUP"() -> (w467:i16)
            n610 = global write "Global_Telescopio.vi" "Estado CUP"("statCUP") -> ()
            n611 = Equal To 0?(x=w465) -> (x = 0?=w464:bool)
            n612 = And(x=w464, y=w449) -> (x .and. y?=w460:bool)
            n613 = case shown="7" "statCUP" {
              selector: "statCUP" -> [w488 _ _ _ _ _ _ _]
              tunnel: [w488 w492 w539 1 w549 w570 w580 w598] -> w453
              tunnel: w469 -> [_ w494 _ _ w551 _ w576 _]
              tunnel: w468 -> [_ w498 _ _ _ _ _ _]
              tunnel: w467 -> [_ w493 _ _ _ _ _ _]
              tunnel: w466 -> [_ w496 _ _ _ _ _ _]
              frame 0, Default {
                # "Sem movimento"
                n614 = call "TickTimeout.vi"() -> ("msTick"=→"TimeoutCUP":u32)  [unwired: 2 in, 2 out]
              }
              frame 1 {
                # "Envia\nComando"
                n615 = local read "LedPointing"() -> (w489:bool)
                n616 = local read "DOME"() -> (w490:bool)
                n617 = Subtract(x=w493, y=w498) -> (x-y=w497:i16)
                n618 = Absolute Value(x=w497) -> (abs(x)=w499:i16)
                n619 = Less Or Equal?(x=w499, y=w496) -> (x <= y?=w495:bool)
                n620 = case shown="True" w495 {
                  tunnel: w494 -> [w505 w529]
                  tunnel: w493 -> [w504 _]
                  tunnel: [w503 w530] -> w492
                  tunnel: "ChkDomeEnable" -> [w500 w528]
                  tunnel: w490 -> [w502 w527]
                  tunnel: w489 -> [w501 w526]
                  frame False {
                    # "CUP fora pos."
                    n621 = case shown="False" w505 {
                      tunnel: w504 -> [w512 _]
                      tunnel: [w510 w520] -> w503
                      tunnel: w502 -> [w509 _]
                      tunnel: w501 -> [w507 _]
                      tunnel: w500 -> [w506 _]
                      frame False {
                        # "CLP Pronto"
                        n622 = Number To Decimal String(number=w512) -> (decimal integer string=w511:string)  [unwired: 1 in]
                        n623 = Select(t=w506, s=w507, f=w509) -> (s? t:f=w508:bool)
                        n624 = case shown="False" w508 {
                          tunnel: [0 2] -> w510
                          tunnel: w511 -> [_ w515]
                          frame False {
                            # "Cúpula Desabilitada"
                            # "Também não verifica\nTrapeira e Paravento"
                          }
                          frame True {
                            w517 = u16 4 items=["ZERO", "AH", "DEC", "TUBO", "CUP"] ("Controlador")
                            n625 = call "TickTimeout.vi"() -> ("msTick"=w514:u32)  [unwired: 2 in, 2 out]
                            n626 = local write "TimeoutCUP"(w514) -> ()
                            n627 = global write "Global_Telescopio.vi" "T cup"(w514) -> ()
                            n628 = call "Monta Comando.vi"("Set Point"=w515, "Comando"="MOVER", "Dispositivo"="DOMO" ("Comando"), "Controlador"=w517) -> ()  [unwired: 3 in, 3 out]
                          }
                        }
                      }
                      frame True {
                        # "CLP Busy"
                        n629 = local read "TimeoutCUP"() -> (w522:u32)
                        n630 = call "TickTimeout.vi"("msInicial"=w522, "msTimeout"=u32 5000) -> ("Timeout"=w521:bool)  [unwired: 2 out]
                        n631 = case shown="True" w521 {
                          tunnel: [1 3] -> w520
                          frame False {
                          }
                          frame True {
                          }
                        }
                      }
                    }
                  }
                  frame True {
                    # "CUP no destino"
                    n632 = case shown="True" w526 {
                      tunnel: [0 w534] -> w530
                      tunnel: w529 -> [_ _]
                      tunnel: w528 -> [_ w533]
                      tunnel: w527 -> [w531 _]
                      frame False {
                        # "Não está apontando (chave Dome Enable foi ativada)"
                        # "Não verifica\nTrapeira e\nParavento"
                        n633 = local write "Dome on Target"(w531) -> ()
                      }
                      frame True {
                        # "Está apontando"
                        n634 = case shown="True" w533 {
                          tunnel: [0 4] -> w534
                          frame False {
                            # "Não verifica\nTrapeira e\nParavento"
                          }
                          frame True {
                            # "Verifica Trapeira e\nParavento"
                            n635 = call "TickTimeout.vi"() -> ("msTick"=w536:u32)  [unwired: 2 in, 2 out]
                            n636 = local write "TimeoutCUP"(w536) -> ()
                            n637 = global write "Global_Telescopio.vi" "T cup"(w536) -> ()
                          }
                        }
                      }
                    }
                  }
                }
              }
              frame 2 {
                w538 = u16 12 items=["Alarme", "Atencao", "Erro", "Ocupado", "TBD", "LCB", "Trapeira", "Paravento", "DomoRap", "DomoCW", "DomoCCW", "TBD", "Em movimento", "TBD"] ("NomeStatus")
                # "Aqui também caberia um Timeout?"
                # "Aguarda parada motor"
                n638 = call "Bit Status CUP.vi"("NomeStatus"=w538) -> ("StatBit"=w540:bool)
                n639 = case shown="True" w540 {
                  tunnel: [1 2] -> w539
                  frame False {
                    # "Motor parado.\nTestar se chegou\nao destino"
                    n640 = call "TickTimeout.vi"() -> ("msTick"=w541:u32)  [unwired: 2 in, 2 out]
                    n641 = local write "TimeoutCUP"(w541) -> ()
                    n642 = global write "Global_Telescopio.vi" "T cup"(w541) -> ()
                  }
                  frame True {
                    # "Ainda movendo...\nAGUARDAR"
                  }
                }
              }
              frame 3 {
                w547 = u16 4 items=["ZERO", "AH", "DEC", "TUBO", "CUP"] ("Controlador")
                # "Trata Timeout"
                n643 = call "TickTimeout.vi"() -> ("msTick"=w544:u32)  [unwired: 2 in, 2 out]
                n644 = local write "TimeoutCUP"(w544) -> ()
                n645 = global write "Global_Telescopio.vi" "T cup"(w544) -> ()
                n646 = call "Monta Comando.vi"("Comando"="PARAR", "Dispositivo"="PROG" ("Comando"), "Controlador"=w547) -> ()  [unwired: 4 in, 3 out]
              }
              frame 4 {
                w550 = u16 7 items=["Alarme", "Atencao", "Erro", "Ocupado", "TBD", "LCB", "Trapeira", "Paravento", "DomoRap", "DomoCW", "DomoCCW", "TBD", "Em movimento", "TBD"] ("NomeStatus")
                # "Verifica Paravento"
                n647 = call "Bit Status CUP.vi"("NomeStatus"=w550) -> ("StatBit"=w554:bool)
                n648 = Not(x=w554) -> (.not. x?=w555:bool)
                n649 = And(x=w555, y="ChkWindDown") -> (x .and. y?=w552:bool)
                n650 = case shown="True" w552 {
                  tunnel: w551 -> [_ w558]
                  tunnel: [6 w557] -> w549
                  frame False {
                    # "Paravento abaixado\nou desabilitado"
                  }
                  frame True {
                    # "Descer Parav."
                    n651 = case shown="True" w558 {
                      tunnel: [5 w563] -> w557
                      frame False {
                        w562 = u16 4 items=["ZERO", "AH", "DEC", "TUBO", "CUP"] ("Controlador")
                        # "Aguardar abaixa/o Parav."
                        # "CLP Pronto"
                        n652 = call "Monta Comando.vi"("Comando"="DESCER", "Dispositivo"="PARAVENTO" ("Comando"), "Controlador"=w562) -> ()  [unwired: 4 in, 3 out]
                      }
                      frame True {
                        # "CLP Busy"
                        n653 = local read "TimeoutCUP"() -> (w565:u32)
                        n654 = call "TickTimeout.vi"("msInicial"=w565, "msTimeout"=u32 5000) -> ("Timeout"=w564:bool)  [unwired: 2 out]
                        n655 = case shown="True" w564 {
                          tunnel: [4 3] -> w563
                          frame False {
                          }
                          frame True {
                          }
                        }
                      }
                    }
                  }
                }
              }
              frame 5 {
                w569 = u16 7 items=["Alarme", "Atencao", "Erro", "Ocupado", "TBD", "LCB", "Trapeira", "Paravento", "DomoRap", "DomoCW", "DomoCCW", "TBD", "Em movimento", "TBD"] ("NomeStatus")
                # "Aqui também caberia um Timeout?"
                # "Também poderia ser testado o bit \"Em movimento\".\nNeste caso o código do \"IF\" deve ser permutado."
                # "Aguarda abaixamento Paravento"
                n656 = call "Bit Status CUP.vi"("NomeStatus"=w569) -> ("StatBit"=w571:bool)
                n657 = case shown="True" w571 {
                  tunnel: [5 6] -> w570
                  frame False {
                    # "Ainda movendo...\nAGUARDAR"
                  }
                  frame True {
                    # "Paravento abaixado."
                  }
                }
              }
              frame 6 {
                w574 = u16 6 items=["Alarme", "Atencao", "Erro", "Ocupado", "TBD", "LCB", "Trapeira", "Paravento", "DomoRap", "DomoCW", "DomoCCW", "TBD", "Em movimento", "TBD"] ("NomeStatus")
                # "Verifica Trapeira"
                n658 = call "Bit Status CUP.vi"("NomeStatus"=w574) -> ("StatBit"=w575:bool)
                n659 = Not(x=w575) -> (.not. x?=w579:bool)
                n660 = And(x=w579, y="ChkOpenShutter") -> (x .and. y?=w577:bool)
                n661 = case shown="True" w577 {
                  tunnel: [0 w584] -> w580
                  tunnel: w576 -> [_ w585]
                  frame False {
                    # "Verificar Paravento"
                    # "Trapeira aberta\nou desabilitada"
                    n662 = call "TickTimeout.vi"() -> ("msTick"=w581:u32)  [unwired: 2 in, 2 out]
                    n663 = local write "TimeoutCUP"(w581) -> ()
